vi "on screen KeyPad.vi"(8 "error in":errorcluster, 11 "Max Value":dbl=5000000.0) -> (0 "error out":errorcluster, 3 "Number out":i32)   [LabVIEW 2015]
panel:
  in  "Number":i32
  in  "Keys":T1
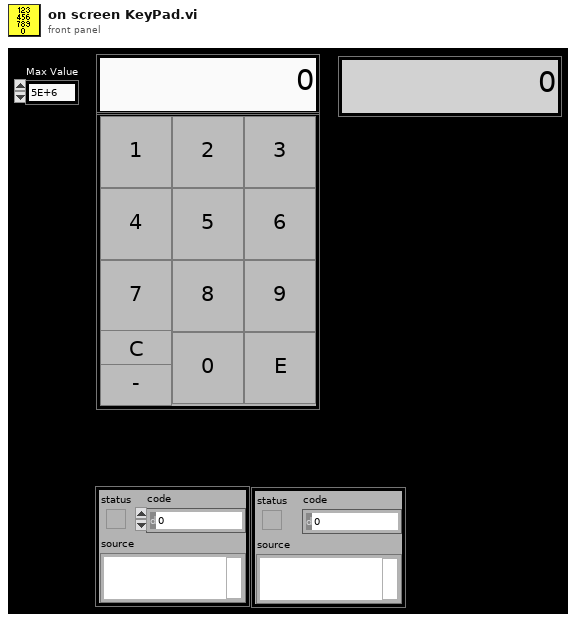
[diagram p1: front panel]
types:
  T1 = cluster{"0":bool, "1":bool, "2":bool, "3":bool, "4":bool, "5":bool, "6":bool, "7":bool, "8":bool, "9":bool, "10":bool, "11":bool, "10 2":bool}
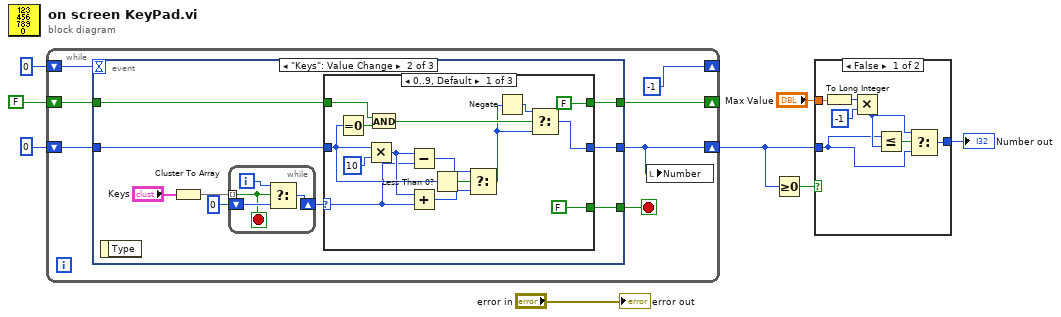
[diagram p0: block diagram]
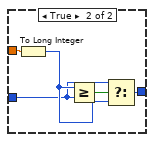
[diagram p2: hidden frame]
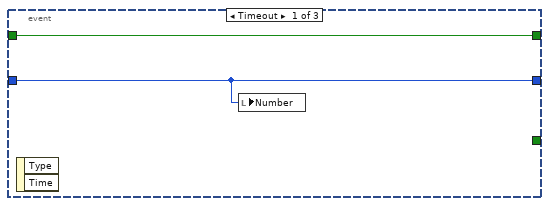
[diagram p3: hidden frame]
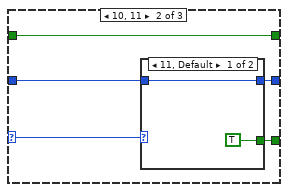
[diagram p4: hidden frame]
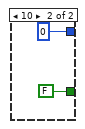
[diagram p5: hidden frame]
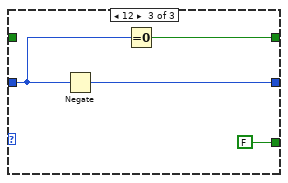
[diagram p6: hidden frame]
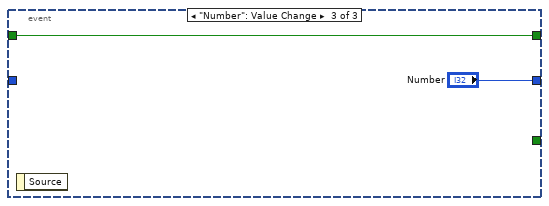
[diagram p7: hidden frame]
diagram:
  n1 = while {
    shift-right: [w11] -> w4
    shift-left: 0 ("Number") -> [w15]
    shift-right: [-1] -> _
    shift-left: 0 -> [w13]
    shift-right: [w9] -> _
    shift-left: FALSE -> [w10]
    stop <- w14 stop-if-true
    n2 = event shown="[1] \"Keys\": Value Change" {
      selector: _ -> [_ _ _]
      dyn-events: _ -> [_ _ _]
      timeout: w13 -> [_ _ _]
      tunnel: w15 -> [w17 w21 _]
      tunnel: [w17 w20 "Number"] -> w11
      tunnel: [_ w22 _] -> w14
      tunnel: w10 -> [w16 w19 w59]
      tunnel: [w16 w18 w59] -> w9
      event Timeout {
        n3 = event-data() -> ()  [unwired: 3 out]
        n4 = local write "Number"(w17) -> ()
      }
      event "Keys": Value Change {
        n5 = event-data() -> ()  [unwired: 2 out]
        n6 = Cluster To Array(cluster="Keys") -> (array=w25:bool[])
        n7 = while {
          tunnel: w25 -> [w55] mode=indexing
          shift-right: [w56] -> w23
          shift-left: 0 ("Number") -> [w58]
          i -> [w57]
          stop <- w55 stop-if-true
          n8 = Select(t=w57, s=w55, f=w58) -> (s? t:f=w56:i32)
        }
        n9 = case shown="0..9, Default" w23 {
          selector: w23 -> [w28 w46 _]
          tunnel: [FALSE w45 FALSE] -> w22
          tunnel: w21 -> [w33 w44 w52]
          tunnel: [w34 w43 w51] -> w20
          tunnel: w19 -> [w38 w42 _]
          tunnel: [FALSE w42 w53] -> w18
          frame 0..9, Default {
            n10 = Equal To 0?(x=w33) -> (x = 0?=w39:bool)
            n11 = Multiply(x=w33, y=10) -> (x*y=w29:i32)
            n12 = And(x=w38, y=w39) -> (x .and. y?=w37:bool)
            n13 = Subtract(x=w29, y=w28) -> (x-y=w27:i32)
            n14 = Add(x=w29, y=w28) -> (x+y=w31:i32)
            n15 = Less Than 0?(x=w33) -> (x < 0?=w32:bool)
            n16 = Select(t=w27, s=w32, f=w31) -> (s? t:f=w30:i32)
            n17 = Negate(x=w30) -> (-x=w35:i32)
            n18 = Select(t=w35, s=w37, f=w30) -> (s? t:f=w34:i32)
          }
          frame 10, 11 {
            n19 = case shown="11, Default" w46 {
              tunnel: [TRUE FALSE] -> w45
              tunnel: [w47 0] -> w43
              tunnel: w44 -> [w47 _]
              frame 11, Default {
              }
              frame 10 {
              }
            }
          }
          frame 12 {
            n20 = Negate(x=w52) -> (-x=w51:i32)
            n21 = Equal To 0?(x=w52) -> (x = 0?=w53:bool)
          }
        }
      }
      event "Number": Value Change {
        n22 = event-data() -> ()  [unwired: 2 out]
      }
    }
    n23 = local write "Number"(w11) -> ()
  }
  n24 = Greater Or Equal To 0?(x=w4) -> (x >= 0?=w3:bool)
  n25 = case shown="False" w3 {
    tunnel: "Max Value" -> [w67 w71]
    tunnel: [w66 w69] -> w2
    tunnel: w4 -> [w61 w68]
    frame False {
      n26 = To Long Integer(number=w67) -> (32bit integer=w65:i32)
      n27 = Multiply(x=w65, y=-1) -> (x*y=w62:i32)
      n28 = Less Or Equal?(x=w61, y=w62) -> (x <= y?=w63:bool)
      n29 = Select(t=w62, s=w63, f=w61) -> (s? t:f=w66:i32)
    }
    frame True {
      n30 = To Long Integer(number=w71) -> (32bit integer=w70:i32)
      n31 = Greater Or Equal?(x=w70, y=w68) -> (x >= y?=w72:bool)
      n32 = Select(t=w68, s=w72, f=w70) -> (s? t:f=w69:i32)
    }
  }
  "Number out" <- w2
  "error out" <- "error in"
